vi "Terminal_Loading_Unit_Display.vi"   [LabVIEW 2014]
types:
  T1 = cluster{"径向油缸加载压力":u16, "轴向油缸加载压力":u16, "油箱1油液温度":u16, "润滑油温度":u16, "油箱2油液温度":u16, "试验轴承供油压力":u16, "试验轴承供油流量":u16, "陪试轴承供油流量":u16, "陪试轴承供油压力":u16, "陪试轴承供油温度":u16, "液压子系统状态字":cluster{"加载单元":cluster{"供油过滤器堵塞报警":bool, "回油过滤器堵塞报警":bool, "液位过高报警":bool, "液位过低报警":bool}, "试验轴承单元":cluster{"加热装置异常报警":bool, "油箱1液位过高报警":bool, "油箱1液位过低报警":bool, "油箱2液位过高报警":bool, "油箱2液位过低报警":bool, "供油过滤器堵塞报警":bool, "循环回路过滤器堵塞报警":bool, "回油过滤器堵塞报警":bool}, "陪试轴承单元":cluster{"供油过滤器1堵塞报警":bool, "供油过滤器2堵塞报警":bool, "回油过滤器堵塞报警":bool, "油箱液位过高报警":bool, "油箱液位过低报警":bool}}}
  T2 = cluster{"供油过滤器堵塞报警":bool, "回油过滤器堵塞报警":bool, "液位过高报警":bool, "液位过低报警":bool}
  T3 = cluster{cluster{sgl, sgl, "径向油缸加载压力":u16}, cluster{sgl, sgl, "轴向油缸加载压力":u16}, "加载单元":cluster{"供油过滤器堵塞报警":bool, "回油过滤器堵塞报警":bool, "液位过高报警":bool, "液位过低报警":bool}}
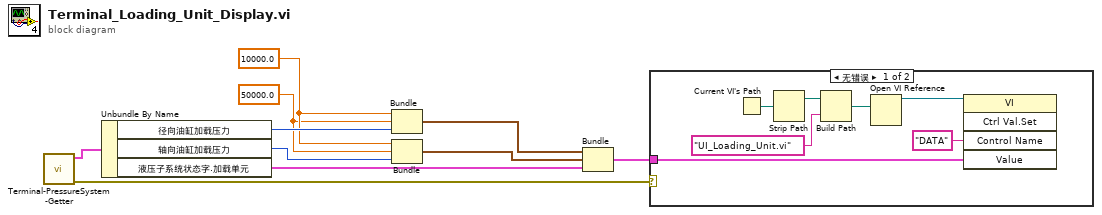
[diagram p0: block diagram]
diagram:
  w8 = sgl 50000.0
  w9 = sgl 10000.0
  n1 = call "Terminal-PressureSystem-Getter.vi"() -> ("error out"=w1:errorcluster, "设备信息"=w3:T1)  [unwired: 10 in]
  n2 = Unbundle By Name(w3) -> ("径向油缸加载压力"=w10:u16, "轴向油缸加载压力"=w7:u16, "液压子系统状态字.加载单元"=w4:T2)
  n3 = Bundle(w9, w8, "径向油缸加载压力"=w10) -> (w6:cluster{sgl, sgl, "径向油缸加载压力":u16})  [unwired: 1 in]
  n4 = Bundle(w9, w8, "轴向油缸加载压力"=w7) -> (w5:cluster{sgl, sgl, "轴向油缸加载压力":u16})  [unwired: 1 in]
  n5 = Bundle(w6, w5, "加载单元"=w4) -> (w2:T3)  [unwired: 1 in]
  n6 = case shown="无错误" w1 {
    tunnel: w2 -> [w11 _]
    frame No Error {
      n7 = Current VI's Path() -> (path=w15:path)
      n8 = Strip Path(path=w15) -> (stripped path=w16:path)  [unwired: 1 out]
      n9 = Build Path(base path=w16, name or relative path="UI_Loading_Unit.vi") -> (appended path=w13:path)
      n10 = Open VI Reference(vi path=w13) -> (vi reference=w12:refnum<vi>)  [unwired: 5 in, 1 out]
      n11 = invoke class="VI" method="Ctrl Val.Set"(reference=w12, "Control Name"="DATA", "Value"=w11) -> ()  [unwired: 2 in, 5 out]
    }
    frame Error {
    }
  }
